vi "Histogram Main.vi"() -> ()   [LabVIEW 2012]
uses:
  Consumer Message.ctl
panel:
  out "Waveform Chart":dbl[](graph)
  in  "Snapshot":bool
  out "Histogram":cluster{"histogram":dbl[], "x axis":dbl[]}(graph)
  out "Consumer Shutdown?":bool
  in  "Stop":bool
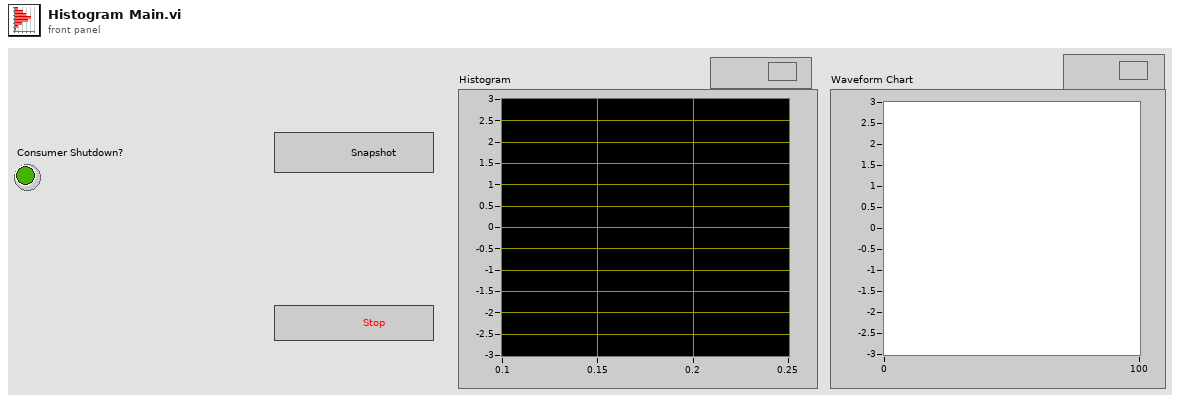
[diagram p1: front panel]
types:
  T1 = typedef "Consumer Message.ctl" = cluster{"Consumer State":string, "Boolean Data":bool, "Numeric Data":i32, "Signal":dbl[], "Error":errorcluster}
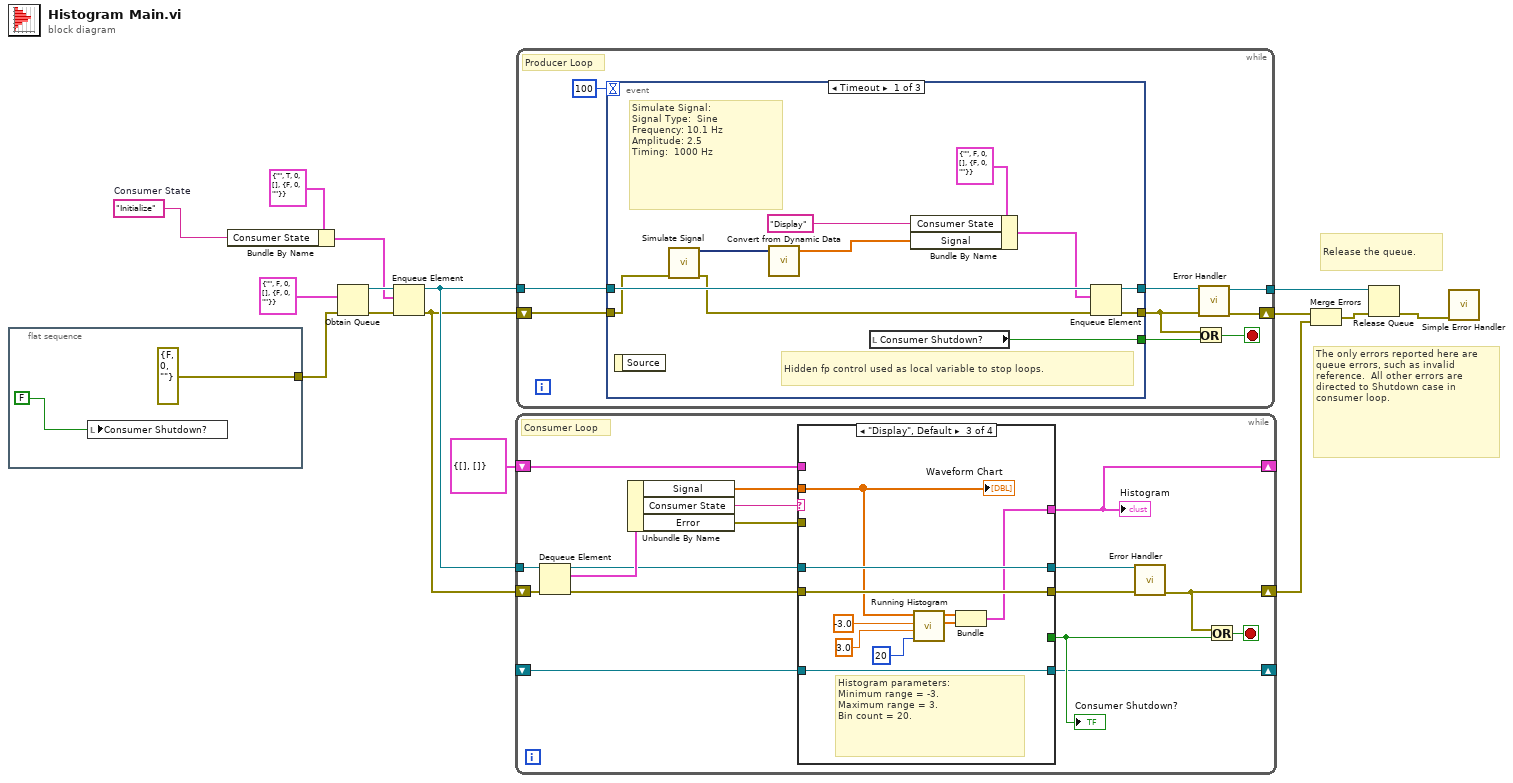
[diagram p0: block diagram]
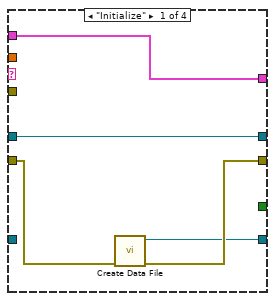
[diagram p2: hidden frame]
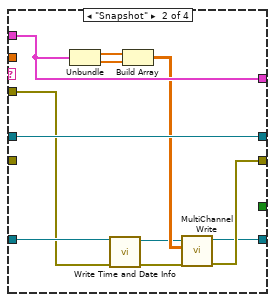
[diagram p3: hidden frame]
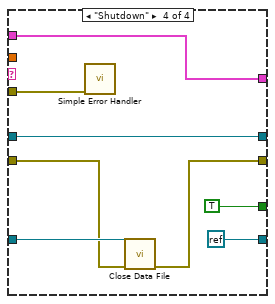
[diagram p4: hidden frame]
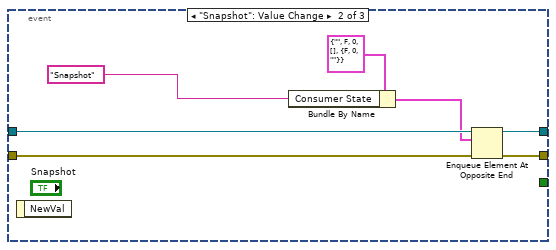
[diagram p5: hidden frame]
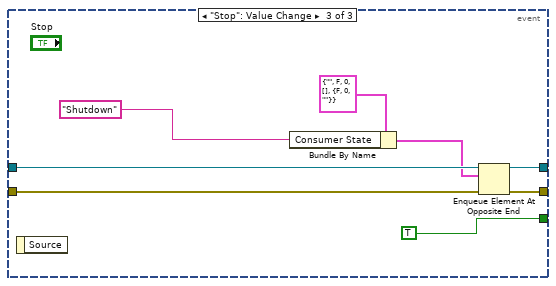
[diagram p6: hidden frame]
diagram:
  w8 = "Initialize"  # Consumer State
  # "Release the queue."
  # "The only errors reported here are queue errors, such as invalid reference.  All other errors are directed to Shutdown case in consumer loop."
  n1 = flat-sequence {
    tunnel: [errorcluster {"status"=FALSE, "code"=0, "source"=""} ("error in (no error)")] -> w11
    frame #0 {
      n2 = local write "Consumer Shutdown?"(FALSE ("Stop Loops (local)")) -> ()
    }
  }
  n3 = Bundle By Name(cluster=T1 {"Consumer State"="", "Boolean Data"=TRUE, "Numeric Data"=0, "Signal"=[], "Error"={"status"=FALSE, "code"=0, "source"=""}} ("Consumer Message"), "Consumer State"=w8) -> (w9:T1)
  n4 = Obtain Queue(element data type=T1 {"Consumer State"="", "Boolean Data"=FALSE, "Numeric Data"=0, "Signal"=[], "Error"={"status"=FALSE, "code"=0, "source"=""}}, error in (no error)=w11) -> (queue out=w13:refnum<queue>, error out=w15:errorcluster)  [unwired: 3 in, 1 out]
  n5 = Enqueue Element(queue=w13, element=w9, error in (no error)=w15) -> (queue out=w12:refnum<queue>, error out=w2:errorcluster)  [unwired: 1 in, 1 out]
  n6 = while {
    tunnel: w12 -> [w34]
    shift-right: [w25] -> w6
    shift-left: w2 -> [w33]
    shift-right: [w18] -> _
    shift-left: cluster{"histogram":dbl[], "x axis":dbl[]} {"histogram"=[], "x axis"=[]} -> [w22]
    shift-right: [w19] -> _
    shift-left: _ -> [w20]
    stop <- w26 stop-if-true
    # "Consumer Loop"
    n7 = Dequeue Element(queue=w34, error in (no error)=w33) -> (queue out=w24:refnum<queue>, element=w32:T1, error out=w23:errorcluster)  [unwired: 1 in, 1 out]
    n8 = Unbundle By Name(w32) -> ("Signal"=w21:dbl[], "Consumer State"=w31:string, "Error"=w28:errorcluster)
    n9 = case shown="\"Display\", Default" w31 {
      tunnel: [_ _ _ TRUE] -> w27
      tunnel: w23 -> [w37 _ w59 w63]
      tunnel: [w36 w46 w59 w62] -> w30
      tunnel: w24 -> [w39 w50 w60 w66]
      tunnel: [w39 w50 w60 w66] -> w29
      tunnel: w28 -> [_ w40 _ w67]
      tunnel: [w38 w48 w56 w65] -> w18
      tunnel: w22 -> [w38 w48 _ w65]
      tunnel: w21 -> [_ _ w54 _]
      tunnel: w20 -> [_ w41 w55 w64]
      tunnel: [w35 w45 w55 refnum<k0> refnum] -> w19
      frame "Initialize" {
        n10 = call "Create Data File.vi"("Error In"=w37) -> ("Error Out"=w36:errorcluster, "File Refnum"=w35:refnum<file>)  [unwired: 9 in]
      }
      frame "Snapshot" {
        n11 = Unbundle(w48) -> ("histogram"=w44:dbl[], "x axis"=w49:dbl[])
        n12 = call "Write Time and Date Info.vi"("Error In"=w40, "File Refnum In"=w41) -> ("Error Out"=w42:errorcluster, "File Refnum Out"=w43:refnum<file>)  [unwired: 6 in]
        n13 = Build Array(w44, w49) -> (w47:dbl[][])
        n14 = call "MultiChannel Write.vi"("Error In"=w42, "Data to Log"=w47, "File Refnum In"=w43) -> ("Error Out"=w46:errorcluster, "File Refnum Out"=w45:refnum<file>)  [unwired: 7 in]
      }
      frame "Display", Default {
        # "Histogram parameters:\nMinimum range = -3.\nMaximum range = 3. \nBin count = 20."
        n15 = call "Running Histogram.vi"("bins"=20, "max"=3.0, "min"=-3.0, "input data"=w54) -> ("x axis"=w57:dbl[], "histogram"=w58:dbl[])  [unwired: 4 in, 2 out]
        n16 = Bundle("histogram"=w58, "x axis"=w57) -> (w56:cluster{"histogram":dbl[], "x axis":dbl[]})  [unwired: 1 in]
        "Waveform Chart" <- w54
      }
      frame "Shutdown" {
        n17 = call <vilib>:"Simple Error Handler.vi"("error in (no error)"=w67) -> ()  [unwired: 4 in, 5 out]
        n18 = call "Close Data File.vi"("error in"=w63, "File Refnum In"=w64) -> ("error out"=w62:errorcluster)  [unwired: 9 in]
      }
    }
    "Consumer Shutdown?" <- w27
    "Histogram" <- w18
    n19 = call "Error Handler.vi"("error in"=w30, "queue in"=w29) -> ("error out"=w25:errorcluster)  [unwired: 8 in, 1 out]
    n20 = Or(x=w25, y=w27) -> (x .or. y?=w26:bool)
  }
  n21 = while {
    tunnel: w12 -> [w77]
    shift-right: [w70] -> w7
    shift-left: w2 -> [w76]
    tunnel: [w69] -> w1
    stop <- w72 stop-if-true
    # "Producer Loop"
    n22 = event shown="[0] Timeout" {
      selector: _ -> [_ _ _]
      dyn-events: _ -> [_ _ _]
      timeout: 100 -> [_ _ _]
      tunnel: w77 -> [w87 w94 w103]
      tunnel: w76 -> [w80 w93 w101]
      tunnel: [w82 w95 w100] -> w71
      tunnel: [w88 _ TRUE] -> w73
      tunnel: [w83 w90 w99] -> w75
      event Timeout {
        # "Simulate Signal:\nSignal Type:  Sine\nFrequency: 10.1 Hz\nAmplitude: 2.5\nTiming:  1000 Hz"
        # "Hidden fp control used as local variable to stop loops."
        n23 = event-data() -> ()  [unwired: 1 in, 1 out]
        n24 = call "Simulate Signal"("error in (no error)"=w80) -> ("Sine with Uniform Noise"=w78:dynamicdata, "error out"=w79:errorcluster)  [unwired: 13 in]
        n25 = call "Convert from Dynamic Data"("Dynamic Data Type"=w78) -> ("Array"=w81:dbl[])  [unwired: 3 in]
        n26 = local read "Consumer Shutdown?"() -> (w88:bool)
        n27 = Bundle By Name(cluster=T1 {"Consumer State"="", "Boolean Data"=FALSE, "Numeric Data"=0, "Signal"=[], "Error"={"status"=FALSE, "code"=0, "source"=""}}, "Consumer State"="Display", "Signal"=w81) -> (w85:T1)
        n28 = Enqueue Element(queue=w87, element=w85, error in (no error)=w79) -> (queue out=w83:refnum<queue>, error out=w82:errorcluster)  [unwired: 1 in, 1 out]
      }
      event "Snapshot": Value Change {
        n29 = event-data() -> ()  [unwired: 1 in, 1 out]
        n30 = Bundle By Name(cluster=T1 {"Consumer State"="", "Boolean Data"=FALSE, "Numeric Data"=0, "Signal"=[], "Error"={"status"=FALSE, "code"=0, "source"=""}}, "Consumer State"="Snapshot" ("String Data")) -> (w91:T1)
        n31 = Enqueue Element At Opposite End(queue=w94, element=w91, error in (no error)=w93) -> (queue out=w90:refnum<queue>, error out=w95:errorcluster)  [unwired: 1 in, 1 out]
      }
      event "Stop": Value Change {
        n32 = event-data() -> ()  [unwired: 1 in, 1 out]
        n33 = Bundle By Name(cluster=T1 {"Consumer State"="", "Boolean Data"=FALSE, "Numeric Data"=0, "Signal"=[], "Error"={"status"=FALSE, "code"=0, "source"=""}}, "Consumer State"="Shutdown") -> (w96:T1)
        n34 = Enqueue Element At Opposite End(queue=w103, element=w96, error in (no error)=w101) -> (queue out=w99:refnum<queue>, error out=w100:errorcluster)  [unwired: 1 in, 1 out]
      }
    }
    n35 = Or(x=w71, y=w73) -> (x .or. y?=w72:bool)
    n36 = call "Error Handler.vi"("error in"=w71, "queue in"=w75) -> ("error out"=w70:errorcluster, "queue out"=w69:refnum<queue>)  [unwired: 8 in]
  }
  n37 = Merge Errors(w7, w6) -> (w4:errorcluster)
  n38 = Release Queue(queue=w1, error in (no error)=w4) -> (error out=w3:errorcluster)  [unwired: 1 in, 2 out]
  n39 = call <vilib>:"Simple Error Handler.vi"("error in (no error)"=w3) -> ()  [unwired: 4 in, 5 out]
